vi "Read Simulation IMU ID.vi"(7 "Analog Channel":T1=enum."AI 1") -> (8 "gyro ID":string, 10 "success?":bool)   [LabVIEW 2017]
uses:
  <vilib>/Rock Robotics/SystemInterfaces/AI/FPGA_AIGyroChannel.ctl
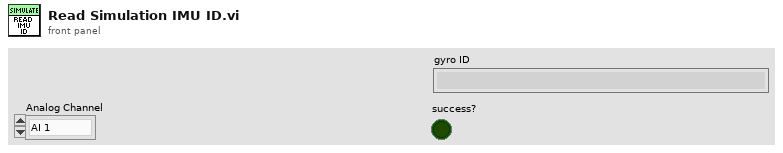
[diagram p1: front panel]
types:
  T1 = typedef "FPGA_AIGyroChannel.ctl" = enum8{"AI 0", "AI 1", "Invalid"}
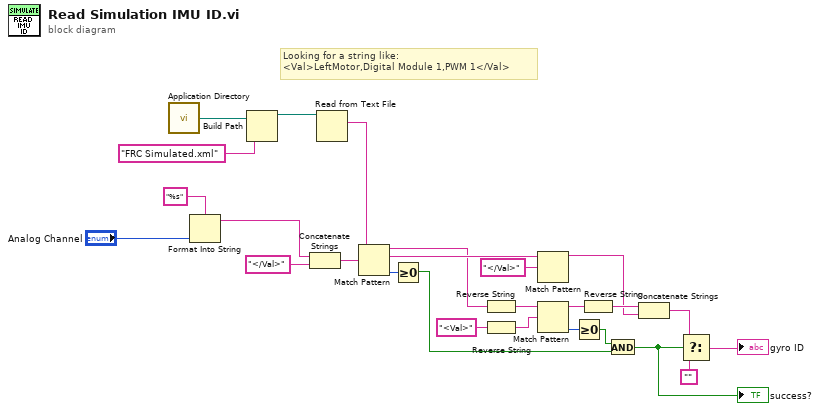
[diagram p0: block diagram]
diagram:
  # "Looking for a string like:\n<Val>LeftMotor,Digital Module 1,PWM 1</Val>"
  n1 = call <vilib>:"Application Directory.vi"() -> ("Application Directory"=w2:path)
  n2 = Format Into String(format string="%s", "Analog Channel") -> (resulting string=w22:string)  [unwired: 2 in, 1 out]
  n3 = Build Path(base path=w2, name or relative path="FRC Simulated.xml") -> (appended path=w20:path)
  n4 = Concatenate Strings(w22, "</Val>" ("name or relative path")) -> (w21:string)
  n5 = Read from Text File(file (use dialog)=w20) -> (text=w24:string)  [unwired: 3 in, 3 out]
  n6 = Match Pattern(string=w24, regular expression=w21) -> (before substring=w11:string, match substring=w15:string, offset past match=w9:i32)  [unwired: 1 in, 1 out]
  n7 = Greater Or Equal To 0?(x=w9) -> (x >= 0?=w7:bool)
  n8 = Reverse String(1:w11) -> (0:w19:string)
  n9 = Reverse String(1:"<Val>" ("name or relative path")) -> (0:w17:string)
  n10 = Match Pattern(string=w15, regular expression="</Val>" ("name or relative path")) -> (before substring=w12:string)  [unwired: 1 in, 3 out]
  n11 = Match Pattern(string=w19, regular expression=w17) -> (before substring=w16:string, offset past match=w10:i32)  [unwired: 1 in, 2 out]
  n12 = Greater Or Equal To 0?(x=w10) -> (x >= 0?=w8:bool)
  n13 = Reverse String(1:w16) -> (0:w13:string)
  n14 = And(x=w8, y=w7) -> (x .and. y?=w6:bool)
  "success?" <- w6
  n15 = Concatenate Strings(w13, w12) -> (w5:string)
  n16 = Select(t=w5, s=w6, f="") -> (s? t:f=→"gyro ID":string)
